vi "Send Force Operation.vi"(8 "error in (no error)":errorcluster, 10 "Force?":bool, 11 "queue in":refnum<queue>) -> (0 "error out":errorcluster, 3 "queue out":refnum<queue>)   [LabVIEW 2016, in "Drive System.lvlib"]
uses:
  Drive System.lvlib
  DriveCmd.ctl
  DriveCmdList.ctl
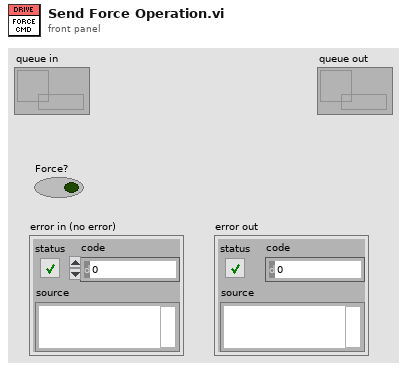
[diagram p1: front panel]
types:
  T1 = typedef "Drive System.lvlib/DriveCmd.ctl" = cluster{"cmd":T2, "data":variant, "Force? (F)":bool, "Lock":string}
  T2 = typedef "Drive System.lvlib/DriveCmdList.ctl" = enum16{"Idle", "Cleanup", "Drive For Time", "Drive Tank", "Drive Arcade", "Unlock", "Lock"}
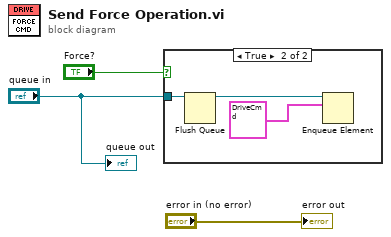
[diagram p0: block diagram]
diagram:
  n1 = case shown="True" "Force?" {
    tunnel: "queue in" -> [_ w6]
    frame False {
    }
    frame True {
      n2 = Flush Queue(queue=w6) -> (queue out=w5:refnum<queue>)  [unwired: 1 in, 2 out]
      n3 = Enqueue Element(queue=w5, element=T1 {"cmd"=enum."Cleanup", "data"=variant, "Force? (F)"=FALSE, "Lock"=""}) -> ()  [unwired: 2 in, 3 out]
    }
  }
  "error out" <- "error in (no error)"
  "queue out" <- "queue in"
